vi "ParaExcel _ Read.vi"(8 "error in":errorcluster) -> (0 "error out":errorcluster, 2 "Units[]":string[](array[string]), 3 "data out":T1(array[cluster]))   [LabVIEW 2016]
uses:
  <vilib>/addons/_office/excel.llb/Excel Get Data ([str]).vi
  <vilib>/Utility/NIReport.llb/NI_report.lvclass
  <vilib>/addons/_office/NI_ReportGenerationToolkit.lvlib
  <vilib>/Utility/NIReport.llb/Excel/NI_Excel.lvclass
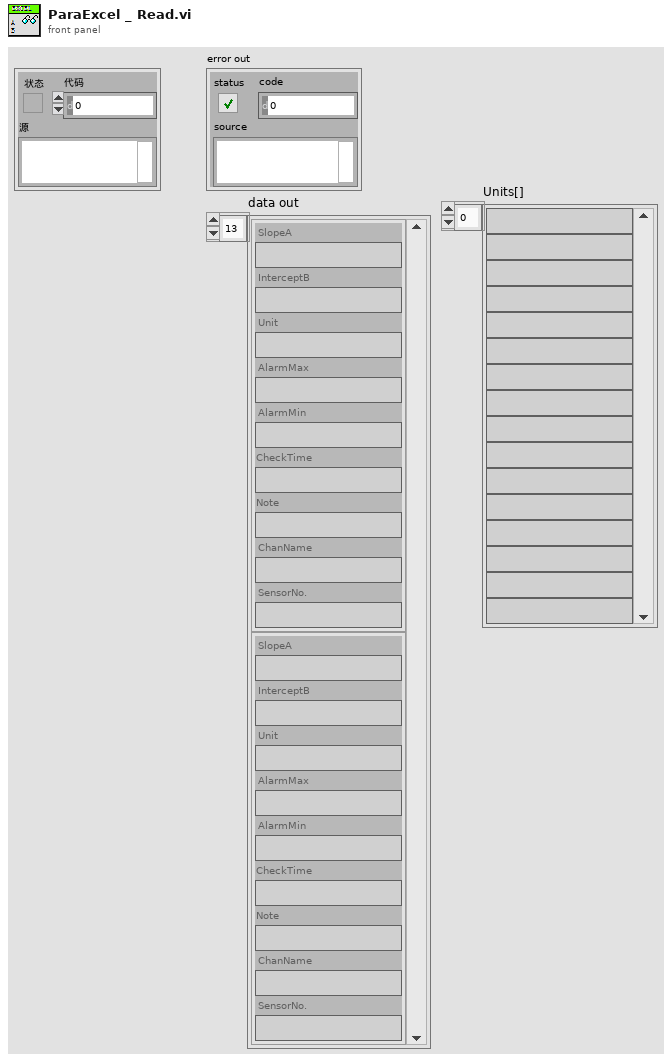
[diagram p1: front panel]
types:
  T1 = cluster{"SlopeA":string, "InterceptB":string, "Unit":string, "AlarmMax":string, "AlarmMin":string, "CheckTime":string, "Note":string, "ChanName":string, "SensorNo.":string}[]
  T2 = enum16{"maximized", "minimized", "normal", "no change"}
  T3 = enum16{"Standard Report", "HTML", "Word", "Excel"}
  T4 = cluster{"output string":string, "output string":string, "trimmed string":string, "output string":string, "output string":string, string, string, string, string}
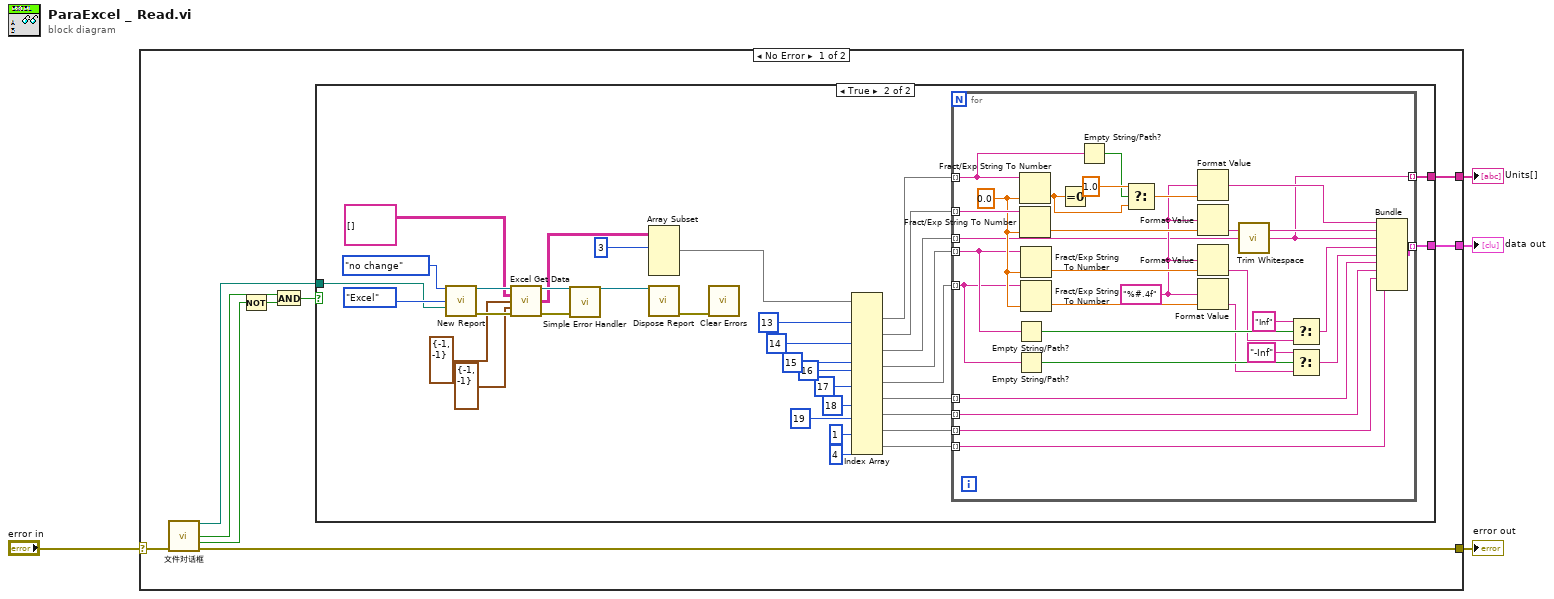
[diagram p0: block diagram]
diagram:
  n1 = case shown="No Error" "error in" {
    selector: "error in" -> [w8 w78]
    tunnel: [w7 _] -> w2
    tunnel: [w6 w78] -> w3
    tunnel: [w5 _] -> w1
    frame No Error {
      n2 = call "文件对话框"("error in"=w8) -> ("selected path"=w9:path, "exists"=w13:bool, "cancelled"=w12:bool, "error out"=w6:errorcluster)  [unwired: 11 in]
      n3 = Not(x=w12) -> (.not. x?=w11:bool)
      n4 = And(x=w13, y=w11) -> (x .and. y?=w10:bool)
      n5 = case shown="True" w10 {
        tunnel: w9 -> [_ w46]
        tunnel: [_ w32] -> w7
        tunnel: [_ w30] -> w5
        frame False {
        }
        frame True {
          n6 = call <vilib>:"New Report.vi"("window state (normal)"=T2."no change", "report type"=T3."Excel", "template (empty)"=w46) -> ("report out"=w26:refnum<class "NI_report.lvclass">, "error out"=w27:errorcluster)  [unwired: 11 in]
          n7 = call-poly <vilib>:"Excel Get Data.vi"("report in"=w26, "data type"=string[][] [], "start (-1, -1)"=cluster{"row":i32, "column":i32} {"row"=-1, "column"=-1}, "end (-1, -1)"=cluster{"row":i32, "column":i32} {"row"=-1, "column"=-1}, "error in (no error)"=w27) -> ("report out"=w23:refnum<class "NI_report.lvclass">, "data"=w20:string[][], "error out"=w21:errorcluster)  [unwired: 8 in]
          n8 = call <vilib>:"Simple Error Handler.vi"("error in (no error)"=w21) -> ()  [unwired: 4 in, 5 out]
          n9 = Array Subset(array=w20, index (row)=3 ("length")) -> (w15:string[][])  [unwired: 3 in]
          n10 = call-dynamic "Dispose Report.vi"("report in"=w23) -> ("error out"=w31:errorcluster)  [unwired: 14 in]
          n11 = call <vilib>:"Clear Errors.vi"("error in (no error)"=w31) -> ()  [unwired: 5 in, 2 out]
          n12 = Index Array(array=w15, index (col) #1=13 ("disabled index (col)"), index (col) #2=14 ("index (col)"), index (col) #3=15 ("index (col)"), index (col) #4=16 ("index (col)"), index (col) #5=17 ("index (col)"), index (col) #6=18 ("index (col)"), index (col) #7=19 ("索引 (列)"), index (col) #8=1 ("index (col)"), index (col) #9=4 ("index (col)")) -> (element #1=w38:string[], element #2=w37:string[], element #3=w36:string[], element #4=w35:string[], element #5=w34:string[], element #6=w33:string[], element #7=w28:string[], element #8=w17:string[], element #9=w16:string[])  [unwired: 9 in]
          n13 = for {
            tunnel: w38 -> [w65] mode=indexing
            tunnel: w37 -> [w77] mode=indexing
            tunnel: w36 -> [w52] mode=indexing
            tunnel: w35 -> [w63] mode=indexing
            tunnel: w34 -> [w57] mode=indexing
            tunnel: w33 -> [w53] mode=indexing
            tunnel: [w74] -> w32 mode=indexing
            tunnel: [w51] -> w30 mode=indexing
            tunnel: w28 -> [w50] mode=indexing
            tunnel: w17 -> [w49] mode=indexing
            tunnel: w16 -> [w48] mode=indexing
            w66 = "%#.4f" ("format string")
            w76 = 0.0 ("default (0 DBL)")
            n14 = Empty String/Path?(string/path=w63) -> (empty?=w62:bool)
            n15 = Empty String/Path?(string/path=w57) -> (empty?=w56:bool)
            n16 = Fract/Exp String To Number(string=w65, default (0 dbl)=w76) -> (number=w72:dbl)  [unwired: 2 in, 1 out]
            n17 = Fract/Exp String To Number(string=w77, default (0 dbl)=w76) -> (number=w67:dbl)  [unwired: 2 in, 1 out]
            n18 = Fract/Exp String To Number(string=w63, default (0 dbl)=w76) -> (number=w69:dbl)  [unwired: 2 in, 1 out]
            n19 = Fract/Exp String To Number(string=w57, default (0 dbl)=w76) -> (number=w75:dbl)  [unwired: 2 in, 1 out]
            n20 = Equal To 0?(x=w72) -> ()  [unwired: 1 out]
            n21 = Empty String/Path?(string/path=w65) -> (empty?=w64:bool)
            n22 = Select(t=1.0, s=w64, f=w72) -> (s? t:f=w68:dbl)
            n23 = Format Value(format string=w66, value (0)=w68) -> (output string=w71:string)  [unwired: 1 in]
            n24 = Format Value(format string=w66, value (0)=w67) -> (output string=w70:string)  [unwired: 1 in]
            n25 = Format Value(format string=w66, value (0)=w69) -> (output string=w60:string)  [unwired: 1 in]
            n26 = Format Value(format string=w66, value (0)=w75) -> (output string=w55:string)  [unwired: 1 in]
            n27 = call <vilib>:"Trim Whitespace.vi"("string"=w52) -> ("trimmed string"=w51:string)  [unwired: 1 in]
            n28 = Select(t="Inf", s=w62, f=w60) -> (s? t:f=w59:string)
            n29 = Select(t="-Inf", s=w56, f=w55) -> (s? t:f=w54:string)
            n30 = Bundle("output string"=w71, "output string"=w70, "trimmed string"=w51, "output string"=w59, "output string"=w54, w53, w50, w49, w48) -> (w74:T4)  [unwired: 1 in]
          }
        }
      }
    }
    frame Error {
    }
  }
  "error out" <- w3
  "data out" <- w2
  "Units[]" <- w1
